vi "Gluelvlchecking.vi"(11 "VISA resource name":refnum<visa-resource-name>) -> (0 "QG":dbl, 3 "VISA resource name out":refnum<visa-resource-name>)   [LabVIEW 2016]
panel:
  out "p":i32
  out "r":i32
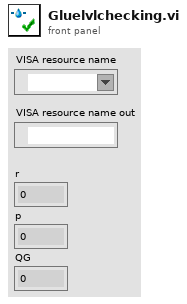
[diagram p1: front panel]
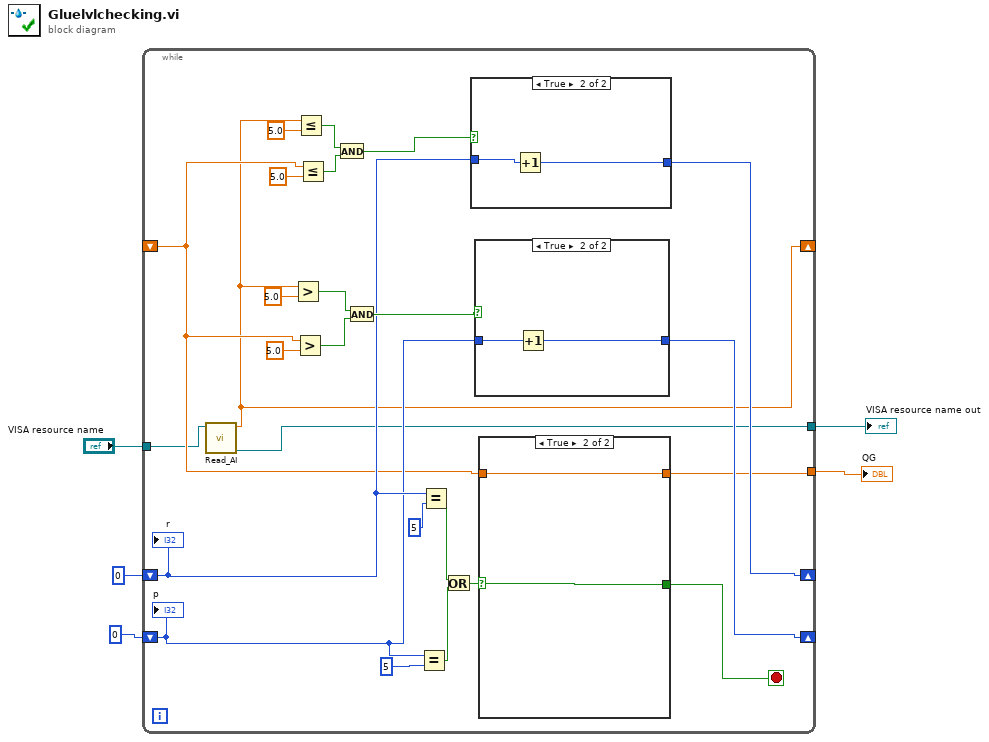
[diagram p0: block diagram]
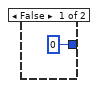
[diagram p3: hidden frame]
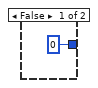
[diagram p4: hidden frame]
diagram:
  n1 = while {
    tunnel: "VISA resource name" -> [w6]
    shift-right: [w8] -> _
    shift-left: _ -> [w14]
    shift-right: [w25] -> _
    shift-left: 0 -> [w18]
    shift-right: [w19] -> _
    shift-left: 0 -> [w17]
    tunnel: [w7] -> w2
    tunnel: [w13] -> w1
    stop <- w9 stop-if-true
    n2 = call "Read_AI.vi"("VISA resource name"=w6) -> ("VISA resource name out"=w7:refnum<visa-resource-name>, "Numeric"=w8:dbl)  [unwired: 9 in]
    n3 = Greater?(x=w8, y=5.0) -> (0:w21:bool)
    n4 = Greater?(x=w14, y=5.0) -> (0:w22:bool)
    n5 = Less Or Equal?(x=w8, y=5.0) -> (x <= y?=w30:bool)
    n6 = Less Or Equal?(x=w14, y=5.0) -> (x <= y?=w29:bool)
    n7 = And(x=w30, y=w29) -> (x .and. y?=w28:bool)
    n8 = And(x=w21, y=w22) -> (x .and. y?=w20:bool)
    n9 = Equal?(x=w17, y=5) -> (x = y?=w11:bool)
    n10 = Equal?(x=w18, y=5) -> (x = y?=w12:bool)
    n11 = Or(x=w12, y=w11) -> (x .or. y?=w10:bool)
    n12 = case shown="True" w28 {
      tunnel: w18 -> [_ w38]
      tunnel: [0 w37] -> w25
      frame False {
      }
      frame True {
        n13 = Increment(x=w38) -> (x+1=w37:i32)
      }
    }
    n14 = case shown="True" w20 {
      tunnel: w17 -> [_ w35]
      tunnel: [0 w34] -> w19
      frame False {
      }
      frame True {
        n15 = Increment(x=w35) -> (x+1=w34:i32)
      }
    }
    n16 = case shown="True" w10 {
      selector: w10 -> [_ w32]
      tunnel: [_ w32] -> w9
      tunnel: w14 -> [_ w31]
      tunnel: [_ w31] -> w13
      frame False {
      }
      frame True {
      }
    }
    "r" <- w18
    "p" <- w17
  }
  "VISA resource name out" <- w2
  "QG" <- w1
